vi "Reverse.vi"() -> ()   [LabVIEW 2014]
uses:
  Robot Global Data.vi
panel:
  in  "Pivot Stick":cluster{"X":dbl, "Y":dbl}
  in  "Wrist Stick":cluster{"Y":dbl, "X":dbl}
  in  "Pivot Multiplier":dbl
  in  "Wrist Multiplier":dbl format="%#_13g"
  out "error out":errorcluster
  in  "error in (no error)":errorcluster
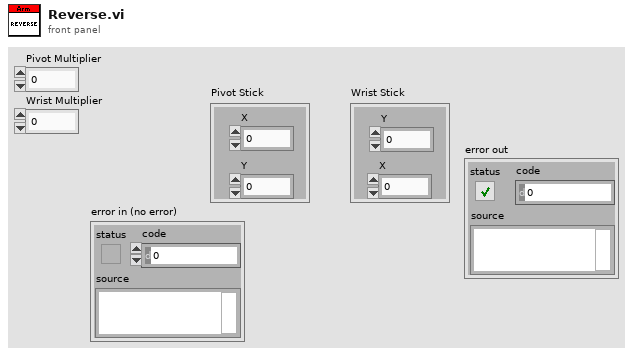
[diagram p1: front panel]
types:
  T1 = typedef "WPI_MotorControlDeviceRef.ctl" = cluster{"DeviceStatus":errorcluster, "Type":T2, "PWM":cluster{"Controller":T3, "PWM Channel":T4, "DeadBand":T5}, "CAN":cluster{"Device Number":u8, "Control Mode":T6, "Semaphore":T7, "Max Vout":dbl, "TalonSRX Control Mode":T8}, "Invert":bool, "TransformRef":T9, "InvTransformRef":T9}
  T2 = typedef "WPI_MotorControlType.ctl" = enum16{"PWM", "CAN", "CANTalonSRX"}
  T3 = typedef "FPGA_TypedefDigitalModule.ctl" = enum16{"Controller 1"}
  T4 = typedef "FPGA_DIOPWMChannel.ctl" = enum8{"PWM 0", "PWM 1", "PWM 2", "PWM 3", "PWM 4", "PWM 5", "PWM 6", "PWM 7", "PWM 8", "PWM 9", "PWM MXP 0", "PWM MXP 1", "PWM MXP 2", "PWM MXP 3", "PWM MXP 4", "PWM MXP 5", "PWM MXP 6", "PWM MXP 7", "PWM MXP 8", "PWM MXP 9", "Invalid"}
  T5 = typedef "WPI_PWMDeadband.ctl" = cluster{"Name":string, "maxPositivePwm":i32, "minPositivePwm":i32, "centerPwm":i32, "maxNegativePwm":i32, "minNegativePwm":i32, "angularRange":u16}
  T6 = typedef "WPI_CANJaguar_ControlMode.ctl" = enum8{"Percent VBus", "Current", "Speed", "Position", "Voltage"}
  T7 = typedef "Semaphore RefNum" = refnum<k1>
  T8 = typedef "WPI_CANTalonSRX_APIControlMode.ctl" = enum8{"Percent VBus", "Speed", "Position", "Slave", "Unchanged / Invalid"}
  T9 = typedef "WPI_PWMTransform_ConPane.ctl" = refnum<vi>
  T10 = typedef "WPI_CANTalonSRX_GlobalStatus.ctl" = cluster{"Applied Throttle":dbl, "Module Enabled":bool, "CAN Error":errorcluster, "Closed Loop Error":dbl, "Forward Limit Switch Closed":bool, "Reverse Limit Switch Closed":bool, "Sensor Position":dbl, "Sensor Velocity":dbl, "Current":dbl, "Sticky Fault - Over Temp":bool, "Sticky Fault - Under Voltage":bool, "Sticky Fault - Forward Limit":bool, "Sticky Fault - Reverse Limit":bool, "Sticky Fault - Forward Soft Limit":bool, "Sticky Fault - Reverse Soft Limit":bool, "Brake is Enabled":bool, "Encoder Position":dbl, "Encoder Velocity":dbl, "Encoder Index Count":dbl, "Encoder A Pin State":bool, "Encoder B Pin State":bool, "Encoder Index Pin State":bool, "Analog In":dbl, "Analog In Velocity":dbl, "Temperature (C)":dbl, "Battery Voltage":dbl}
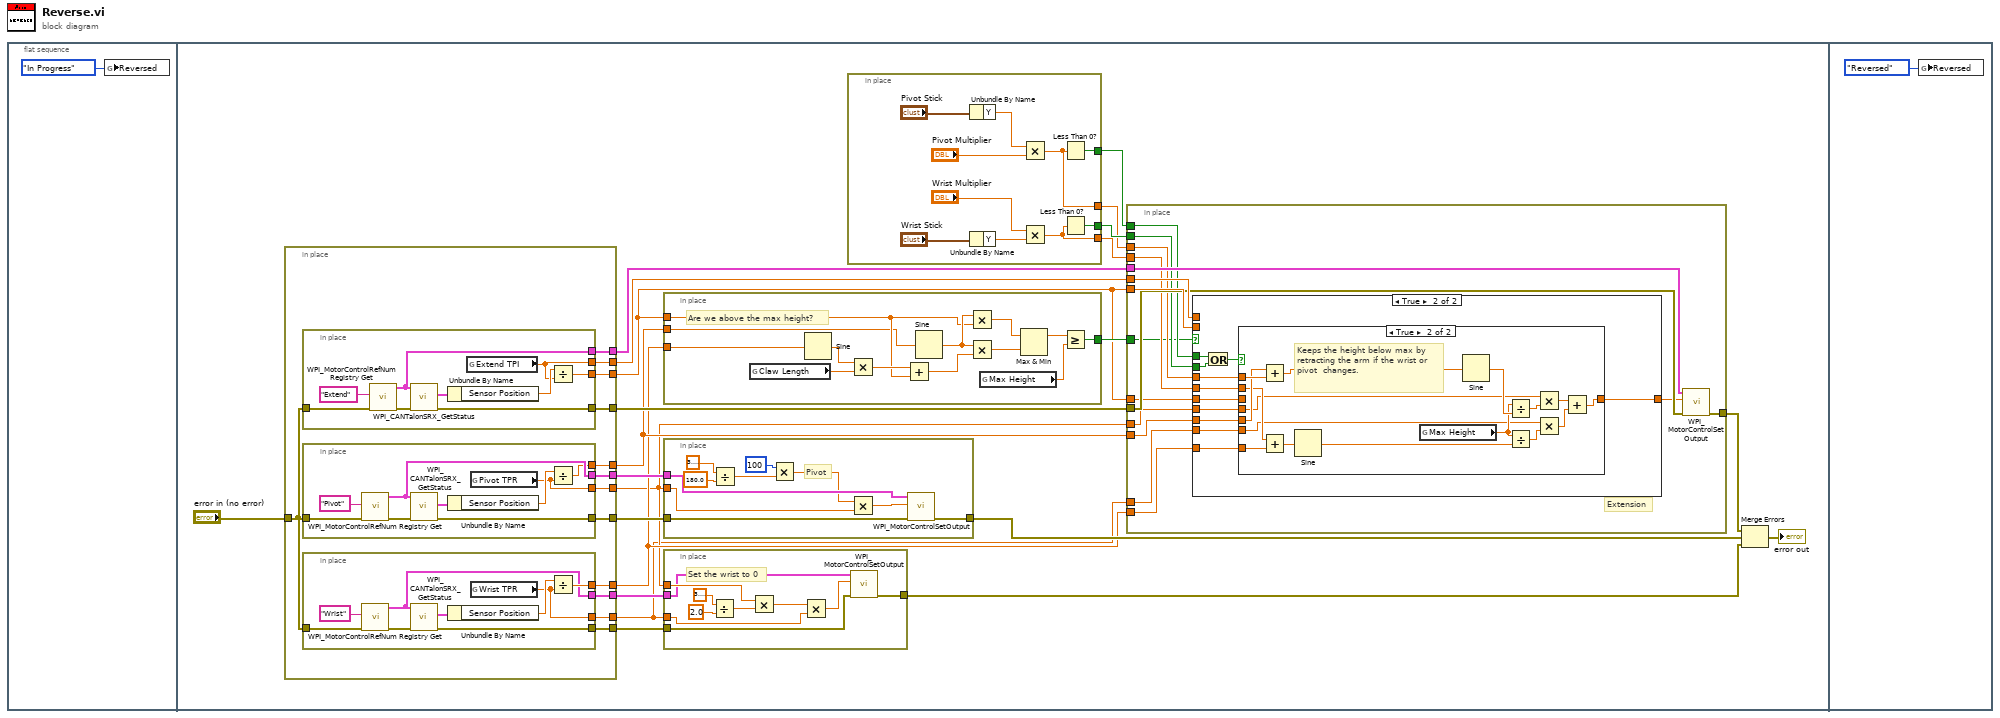
[diagram p0: block diagram]
diagram:
  n1 = flat-sequence {
    frame #0 {
      n2 = global write "Robot Global Data.vi" "Reversed"(enum16{"Normal", "In Progress", "Reversed"}."In Progress" ("Reversed")) -> ()
    }
    frame #1 {
      n3 = in-place {
        in-place-border: "error in (no error)" -> [w101]
        in-place-border: [w100] -> w3
        in-place-border: [w99] -> w20
        in-place-border: [w98] -> w19
        in-place-border: [w97] -> w18
        in-place-border: [w96] -> w17
        in-place-border: [w95] -> w16
        in-place-border: [w94] -> w10
        in-place-border: [w93] -> w4
        in-place-border: [w92] -> w11
        in-place-border: [w91] -> w5
        in-place-border: [w90] -> w13
        in-place-border: [w89] -> w12
        n4 = in-place {
          in-place-border: w101 -> [w110]
          in-place-border: [w105] -> w100
          in-place-border: [w104] -> w99
          in-place-border: [w103] -> w98
          in-place-border: [w102] -> w97
          n5 = call <vilib>:"WPI_MotorControlRefNum Registry Get.vi"("error in (no error)"=w110, "refnum name"="Extend") -> ("error out"=w107:errorcluster, "MotorControlDevRef"=w103:T1)  [unwired: 8 in]
          n6 = call <vilib>:"WPI_CANTalonSRX_GetStatus.vi"("error in (no error)"=w107, "CAN Talon SRX Ref"=w103) -> ("error out"=w102:errorcluster, "Talon SRX Status"=w108:T10)  [unwired: 7 in, 1 out]
          n7 = Unbundle By Name(w108) -> ("Sensor Position"=w106:dbl)
          n8 = global read "Robot Global Data.vi" "Extend TPI"() -> (w104:dbl)
          n9 = Divide(x=w106, y=w104) -> (x/y=w105:dbl)
        }
        n10 = in-place {
          in-place-border: w101 -> [w119]
          in-place-border: [w117] -> w96
          in-place-border: [w116] -> w95
          in-place-border: [w112] -> w92
          in-place-border: [w113] -> w91
          n11 = call <vilib>:"WPI_MotorControlRefNum Registry Get.vi"("error in (no error)"=w119, "refnum name"="Pivot") -> ("error out"=w118:errorcluster, "MotorControlDevRef"=w117:T1)  [unwired: 8 in]
          n12 = call <vilib>:"WPI_CANTalonSRX_GetStatus.vi"("error in (no error)"=w118, "CAN Talon SRX Ref"=w117) -> ("error out"=w116:errorcluster, "Talon SRX Status"=w115:T10)  [unwired: 7 in, 1 out]
          n13 = Unbundle By Name(w115) -> ("Sensor Position"=w114:dbl)
          n14 = global read "Robot Global Data.vi" "Pivot TPR"() -> (w113:dbl)
          n15 = Divide(x=w114, y=w113) -> (x/y=w112:dbl)
        }
        n16 = in-place {
          in-place-border: w101 -> [w127]
          in-place-border: [w125] -> w89
          in-place-border: [w124] -> w94
          in-place-border: [w121] -> w93
          in-place-border: [w120] -> w90
          n17 = call <vilib>:"WPI_MotorControlRefNum Registry Get.vi"("error in (no error)"=w127, "refnum name"="Wrist") -> ("error out"=w126:errorcluster, "MotorControlDevRef"=w120:T1)  [unwired: 8 in]
          n18 = call <vilib>:"WPI_CANTalonSRX_GetStatus.vi"("error in (no error)"=w126, "CAN Talon SRX Ref"=w120) -> ("error out"=w125:errorcluster, "Talon SRX Status"=w128:T10)  [unwired: 7 in, 1 out]
          n19 = Unbundle By Name(w128) -> ("Sensor Position"=w122:dbl)
          n20 = global read "Robot Global Data.vi" "Wrist TPR"() -> (w121:dbl)
          n21 = Divide(x=w122, y=w121) -> (x/y=w124:dbl)
        }
      }
      n22 = in-place {
        in-place-border: [w139] -> w22
        in-place-border: w3 -> [w148]
        in-place-border: w10 -> [w146]
        in-place-border: w11 -> [w145]
        # "Are we above the max height?"
        n23 = global read "Robot Global Data.vi" "Claw Length"() -> (w144:dbl)
        n24 = Sine(x=w146) -> (sin(x)=w147:dbl)
        n25 = Multiply(x=w147, y=w144) -> (x*y=w150:dbl)
        n26 = Add(x=w150, y=w148) -> (x+y=w149:dbl)
        n27 = Sine(x=w145) -> (sin(x)=w151:dbl)
        n28 = Multiply(x=w151, y=w148) -> (x*y=w143:dbl)
        n29 = Multiply(x=w151, y=w149) -> (x*y=w142:dbl)
        n30 = global read "Robot Global Data.vi" "Max Height"() -> (w140:dbl)
        n31 = Max & Min(x=w143, y=w142) -> (max(x,y)=w141:dbl)  [unwired: 1 out]
        n32 = Greater Or Equal?(x=w141, y=w140) -> (x >= y?=w139:bool)
      }
      n33 = in-place {
        in-place-border: w17 -> [w33]
        in-place-border: w16 -> [w32]
        in-place-border: [w31] -> w14
        in-place-border: w5 -> [w24]
        # "Pivot"
        n34 = Divide(x=3.141592653589793, y=180.0 ("x")) -> (x/y=w29:dbl)
        n35 = Multiply(x=100, y=w29) -> (x*y=w25:dbl)
        n36 = Multiply(x=w25, y=w24) -> (x*y=w26:dbl)
        n37 = call <vilib>:"WPI_MotorControlSetOutput.vi"("error in (no error)"=w32, "Output"=w26, "MotorControlDevRef"=w33) -> ("error out"=w31:errorcluster)  [unwired: 6 in, 2 out]
      }
      n38 = in-place {
        in-place-border: w5 -> [w138]
        in-place-border: w13 -> [w137]
        in-place-border: [w136] -> w2
        in-place-border: w12 -> [w135]
        in-place-border: w4 -> [w129]
        # "Set the wrist to 0"
        n39 = Divide(x=3.141592653589793, y=2.0) -> (x/y=w133:dbl)
        n40 = Multiply(x=w138, y=w133) -> (x*y=w131:dbl)
        n41 = Multiply(x=w131, y=w129) -> (x*y=w130:dbl)
        n42 = call <vilib>:"WPI_MotorControlSetOutput.vi"("error in (no error)"=w135, "Output"=w130, "MotorControlDevRef"=w137) -> ("error out"=w136:errorcluster)  [unwired: 6 in, 2 out]
      }
      n43 = in-place {
        in-place-border: [w81] -> w7
        in-place-border: [w79] -> w6
        in-place-border: [w82] -> w9
        in-place-border: [w80] -> w8
        n44 = Unbundle By Name("Pivot Stick") -> ("Y"=w85:dbl)
        n45 = Unbundle By Name("Wrist Stick") -> ("Y"=w84:dbl)
        n46 = Multiply(x=w85, y="Pivot Multiplier") -> (x*y=w81:dbl)
        n47 = Multiply(x="Wrist Multiplier", y=w84) -> (x*y=w79:dbl)
        n48 = Less Than 0?(x=w81) -> (x < 0?=w82:bool)
        n49 = Less Than 0?(x=w79) -> (x < 0?=w80:bool)
      }
      n50 = in-place {
        in-place-border: w22 -> [w35]
        in-place-border: w3 -> [w49]
        in-place-border: w20 -> [w48]
        in-place-border: w19 -> [w47]
        in-place-border: w18 -> [w46]
        in-place-border: [w44] -> w15
        in-place-border: w7 -> [w43]
        in-place-border: w6 -> [w42]
        in-place-border: w11 -> [w41]
        in-place-border: w10 -> [w40]
        in-place-border: w4 -> [w39]
        in-place-border: w5 -> [w38]
        in-place-border: w9 -> [w37]
        in-place-border: w8 -> [w36]
        in-place-border: w3 -> [w34]
        # "Extension"
        n51 = case shown="True" w35 {
          tunnel: w49 -> [_ _]
          tunnel: w48 -> [_ _]
          tunnel: [w50 w52] -> w45
          tunnel: w36 -> [_ w61]
          tunnel: w37 -> [_ w60]
          tunnel: w43 -> [_ w58]
          tunnel: w42 -> [_ w57]
          tunnel: w41 -> [_ w56]
          tunnel: w40 -> [_ w55]
          tunnel: w39 -> [_ w54]
          tunnel: w38 -> [_ w53]
          tunnel: w34 -> [w50 w51]
          frame False {
          }
          frame True {
            n52 = Or(x=w60, y=w61) -> (x .or. y?=w59:bool)
            n53 = case shown="True" w59 {
              tunnel: w58 -> [_ w78]
              tunnel: w57 -> [_ w69]
              tunnel: w56 -> [_ w77]
              tunnel: w55 -> [_ w68]
              tunnel: w54 -> [_ w67]
              tunnel: w53 -> [_ w66]
              tunnel: [w62 w63] -> w52
              tunnel: w51 -> [w62 _]
              frame False {
              }
              frame True {
                # "Keeps the height below max by retracting the arm if the wrist or pivot  changes."
                n54 = Add(x=w77, y=w78) -> (x+y=w76:dbl)
                n55 = Add(x=w69, y=w68) -> (x+y=w73:dbl)
                n56 = Sine(x=w73) -> (sin(x)=w72:dbl)
                n57 = global read "Robot Global Data.vi" "Max Height"() -> (w70:dbl)
                n58 = Sine(x=w76) -> (sin(x)=w75:dbl)
                n59 = Divide(x=w70, y=w75) -> (x/y=w74:dbl)
                n60 = Divide(x=w70, y=w72) -> (x/y=w71:dbl)
                n61 = Multiply(x=w66, y=w74) -> (x*y=w65:dbl)
                n62 = Multiply(x=w67, y=w71) -> (x*y=w64:dbl)
                n63 = Add(x=w65, y=w64) -> (x+y=w63:dbl)
              }
            }
          }
        }
        n64 = call <vilib>:"WPI_MotorControlSetOutput.vi"("error in (no error)"=w46, "Output"=w45, "MotorControlDevRef"=w47) -> ("error out"=w44:errorcluster)  [unwired: 6 in, 2 out]
      }
      n65 = Merge Errors(w15, w14, w2) -> (→"error out":errorcluster)
    }
    frame #2 {
      n66 = global write "Robot Global Data.vi" "Reversed"(enum16{"Normal", "In Progress", "Reversed"}."Reversed" ("Reversed")) -> ()
    }
  }
